vi "example plot from array with titles.vi"() -> ()   [LabVIEW 2009]
panel:
  in  "output array":string[][](array[string])=[["Cam1 shot #", "Cam1 exposure", "Cam1 trigger"], ["-1", "1.000000", "on"], ["-1", "1.000000", "on"], ["-1", "1.000000", "on"], ["-1", "1.000000", "on"], ["-1", "1.000000", "on"], ["-1", "1.000000", "on"], ["-1", "1.000000", "on"]]
  in  "X Axis":u16(ring)=1 items=["Cam1 shot #", "Cam1 exposure", "Cam1 trigger"]
  out "Energy transmission 2":cluster{dbl[], dbl[]}(graph)={[1.0, 1.0, 1.0, 1.0, 1.0, 1.0, 1.0], [-1.0, -1.0, -1.0, -1.0, -1.0, -1.0, -1.0]}
  in  "Y Axis":u16(ring) items=["Cam1 shot #", "Cam1 exposure", "Cam1 trigger"]
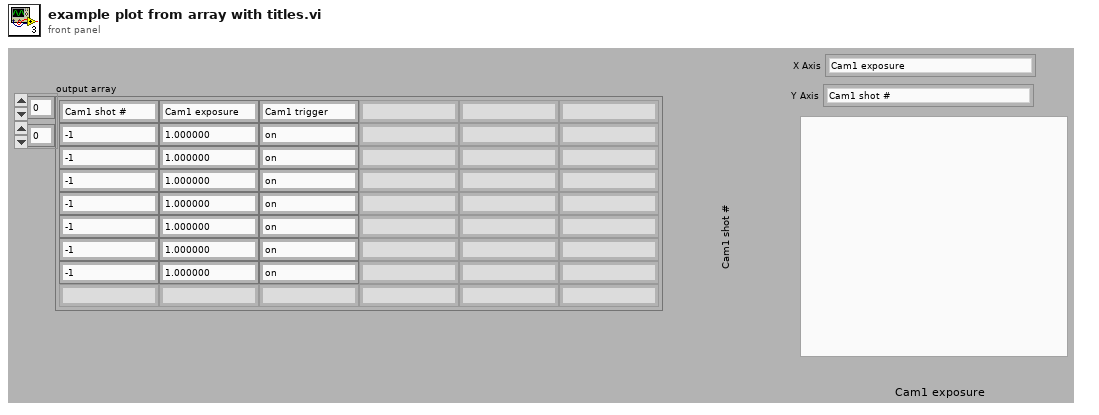
[diagram p1: front panel]
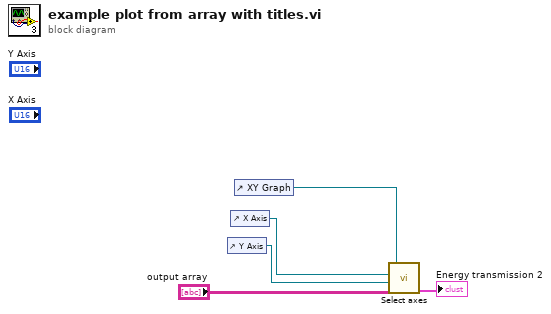
[diagram p0: block diagram]
diagram:
  n1 = control-ref of="Y Axis"() -> (w1:refnum<vi>)
  n2 = control-ref of="X Axis"() -> (w2:refnum<vi>)
  n3 = control-ref of="XY Graph"() -> (w3:refnum<vi>)
  n4 = call "Select axes.vi"("XYGraph Refnum"=w3, "Ring Refnum"=w2, "Ring Refnum 2"=w1, "output array"="output array") -> ("Cluster"=→"Energy transmission 2":cluster{dbl[], dbl[]})  [unwired: 4 out]
